vi "MicroscopyFileNamer.vi"(5 "Location":T1=enum."WCM Main", 6 "Create Folder Now?":bool=TRUE, 7 "String in":string, 8 "FileCount":i32, 9 "Type of scan":T2, 10 "Microscopy Scan Mode":T3(ring), 11 "Save Path In":path) -> (2 "FIle Name out":string, 3 "Scan Data Path":path)   [LabVIEW 2022 SP3]
uses:
  Controls/ScanType2.ctl
  Controls/location.ctl
  Motion Controllers/-MotionRoutines/MotionGlobals.vi
  <vilib>/regexp/Match Regular Expression.xnode
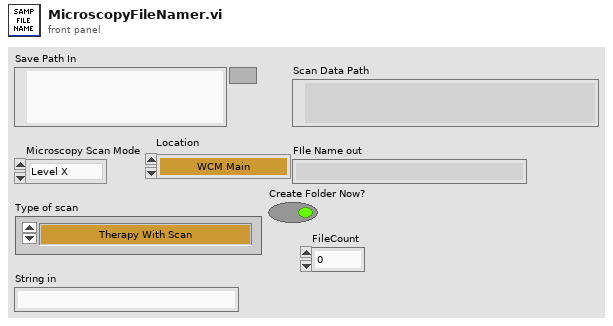
[diagram p1: front panel]
types:
  T1 = typedef "location.ctl" = enum16{"Automatic", "WCM Main", "Hawaii", "Columbia MM3000", "Columbia  NI System", "NYU", "RRI 2", "UHI Allen", "CUMC RT", "Chiba", "Stony Brook", "WCM Microscopy", "WCM Aeoretch", "WCM Optics Lab", "WCM Main 2Axis", "WCM Rotation", "WCM SAM SMAC", "SERI GP"}
  T2 = typedef "ScanType2.ctl" = enum16{"Therapy With Scan", "M scan", "M Scan With Therapy Burst", "1-D B Scan", "1-D B Scan With Therapy Burst", "2-D B Scan", "2-D B Scan With Therapy Burst", "Rotational Scan", "1-D B-Scan PRF", "2-D B-Scan PRF", "Real-Time Scan", "Contrast Agents", "1-D w/ Real-Time Set Up", "Dual Transducer", "Acoustic Microscopy", "Hydrophone Scanning"}
  T3 = enum32{"Level X", "Level Y", "Overview Scan", "Detailed Scan", "V-Z Scan"}
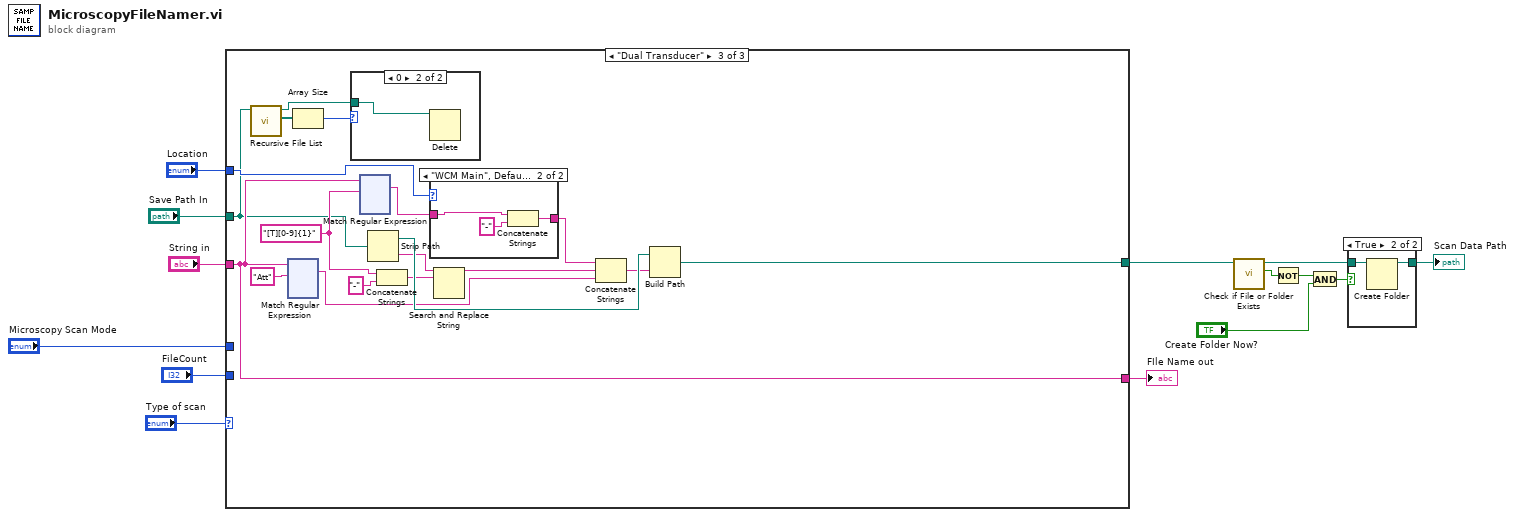
[diagram p0: block diagram]
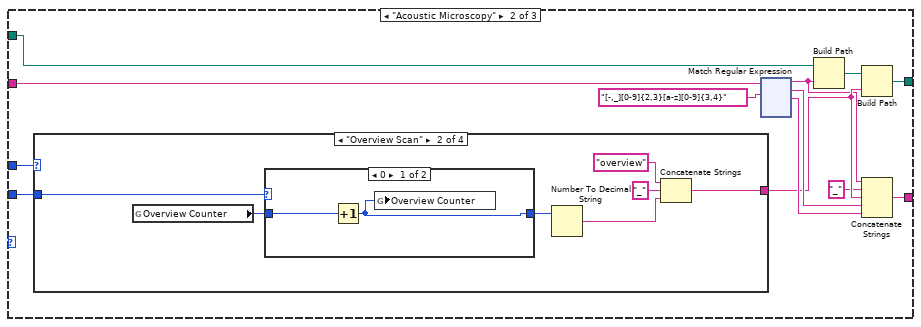
[diagram p4: hidden frame]
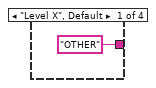
[diagram p5: hidden frame]
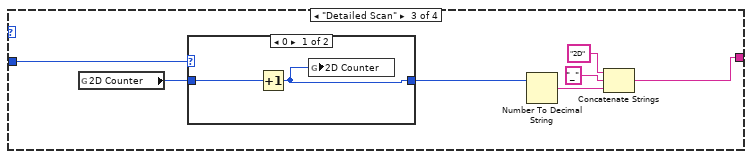
[diagram p7: hidden frame]
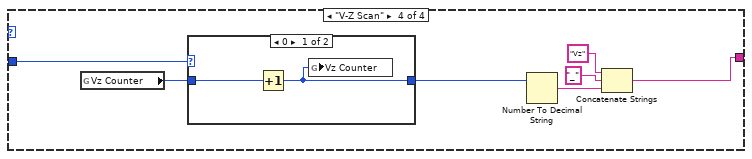
[diagram p9: hidden frame]
diagram:
  n1 = case shown="\"Dual Transducer\"" "Type of scan" {
    tunnel: "String in" -> [w16 w23 w192]
    tunnel: [w16 w26 w192] -> w11
    tunnel: "Microscopy Scan Mode" -> [_ w25 _]
    tunnel: "Save Path In" -> [w15 w24 w181]
    tunnel: [w15 w22 w195] -> w14
    tunnel: "FileCount" -> [_ w17 _]
    tunnel: "Location" -> [_ _ w189]
    frame "Therapy With Scan", Default {
    }
    frame "Acoustic Microscopy" {
      n2 = case shown="\"Overview Scan\"" w25 {
        tunnel: ["OTHER" ("regular expression 2") w36 w44 w52] -> w21
        tunnel: w17 -> [_ w33 w43 w51]
        frame "Level X", Default {
        }
        frame "Overview Scan" {
          n3 = global read "MotionGlobals.vi" "Overview Counter"() -> (w35:i16)
          n4 = case shown="0" w33 {
            tunnel: w35 -> [w39 w40]
            tunnel: [w38 w40] -> w34
            frame 0 {
              n5 = Increment(x=w39) -> (x+1=w38:i16)
              n6 = global write "MotionGlobals.vi" "Overview Counter"(w38) -> ()
            }
            frame 1, Default {
            }
          }
          n7 = Number To Decimal String(number=w34) -> (decimal integer string=w32:string)  [unwired: 1 in]
          n8 = Concatenate Strings("overview" ("regular expression 2"), "_" ("string"), w32) -> (w36:string)
        }
        frame "Detailed Scan" {
          n9 = global read "MotionGlobals.vi" "2D Counter"() -> (w47:i16)
          n10 = case shown="0" w43 {
            tunnel: w47 -> [w49 w50]
            tunnel: [w48 w50] -> w46
            frame 0 {
              n11 = Increment(x=w49) -> (x+1=w48:i16)
              n12 = global write "MotionGlobals.vi" "2D Counter"(w48) -> ()
            }
            frame 1, Default {
            }
          }
          n13 = Number To Decimal String(number=w46) -> (decimal integer string=w42:string)  [unwired: 1 in]
          n14 = Concatenate Strings("2D" ("regular expression 2"), "_" ("string"), w42) -> (w44:string)
        }
        frame "V-Z Scan" {
          n15 = global read "MotionGlobals.vi" "Vz Counter"() -> (w57:i16)
          n16 = case shown="0" w51 {
            tunnel: w57 -> [w59 w60]
            tunnel: [w58 w60] -> w56
            frame 0 {
              n17 = Increment(x=w59) -> (x+1=w58:i16)
              n18 = global write "MotionGlobals.vi" "Vz Counter"(w58) -> ()
            }
            frame 1, Default {
            }
          }
          n19 = Number To Decimal String(number=w56) -> (decimal integer string=w55:string)  [unwired: 1 in]
          n20 = Concatenate Strings("Vz" ("regular expression 2"), "_" ("string"), w55) -> (w52:string)
        }
      }
      n21 = xnode "Match Regular Expression"("input string"=w23, "regular expression"="[-,_][0-9]{2,3}[a-z][0-9]{3,4}" ("regular expression 2")) -> ("before match"=w18:string, "whole match"=w29:string, "after match"=w28:string)  [unwired: 4 in, 2 out]
      n22 = Build Path(base path=w24, name or relative path=w18) -> (appended path=w19:path)
      n23 = Build Path(base path=w19, name or relative path=w21) -> (appended path=w22:path)
      n24 = Concatenate Strings(w18, "_" ("string"), w21, w29, w28) -> (w26:string)
    }
    frame "Dual Transducer" {
      w184 = "[T][0-9]{1}" ("regular expression 2")
      n25 = call <vilib>:"Recursive File List.vi"("Folder Path"=w181) -> ("All Files in Dir"=w180:path[], "dup Folder Path"=w178:path)  [unwired: 6 in, 3 out]
      n26 = xnode "Match Regular Expression"("input string"=w192, "regular expression"="Att") -> ("whole match"=w190:string)  [unwired: 4 in, 4 out]
      n27 = Array Size(array=w180) -> (size(s)=w179:i32)
      n28 = case shown="0" w179 {
        tunnel: w178 -> [_ w196]
        frame 1, Default {
        }
        frame 0 {
          n29 = Delete(path (use dialog)=w196) -> ()  [unwired: 4 in, 3 out]
        }
      }
      n30 = xnode "Match Regular Expression"("input string"=w192, "regular expression"=w184) -> ("whole match"=w187:string)  [unwired: 4 in, 4 out]
      n31 = Strip Path(path=w181) -> (stripped path=w194:path, name=w186:string)
      n32 = Concatenate Strings(w184, "-" ("string")) -> (w183:string)
      n33 = case shown="\"WCM Main\", Default" w189 {
        tunnel: [w197 w199] -> w188
        tunnel: w187 -> [w197 w200]
        frame "Hawaii" {
        }
        frame "WCM Main", Default {
          n34 = Concatenate Strings(w200, "-" ("string")) -> (w199:string)
        }
      }
      n35 = Search and Replace String(input string=w186, search string=w183) -> (result string=w185:string)  [unwired: 6 in, 3 out]
      n36 = Concatenate Strings(w188, w185, w190) -> (w193:string)
      n37 = Build Path(base path=w194, name or relative path=w193) -> (appended path=w195:path)
    }
  }
  "FIle Name out" <- w11
  n38 = call <vilib>:"Check if File or Folder Exists.vi"("path"=w14) -> ("file or folder exists?"=w6:bool, "dup path"=w8:path)  [unwired: 8 in, 1 out]
  n39 = Not(x=w6) -> (.not. x?=w1:bool)
  n40 = And(x=w1, y="Create Folder Now?") -> (x .and. y?=w3:bool)
  n41 = case shown="True" w3 {
    tunnel: w8 -> [w435 w437]
    tunnel: [w435 w436] -> w7
    frame False {
    }
    frame True {
      n42 = Create Folder(path (use dialog)=w437) -> (created path=w436:path)  [unwired: 2 in, 2 out]
    }
  }
  "Scan Data Path" <- w7
